vi "thcd_rest_gets.vi"(2 "thcd_delay":u32=500, 3 "thcd_visa":refnum<visa-resource-name>) -> ()   [LabVIEW 2013]
panel:
  in  "thcd_ch":u8(ring) items=["1"=1, "2"=2, "3"=3, "4"=4, "all"=5]
  in  "thcd_com":T1(ring)
  out "error out":errorcluster
  in  "error in":errorcluster
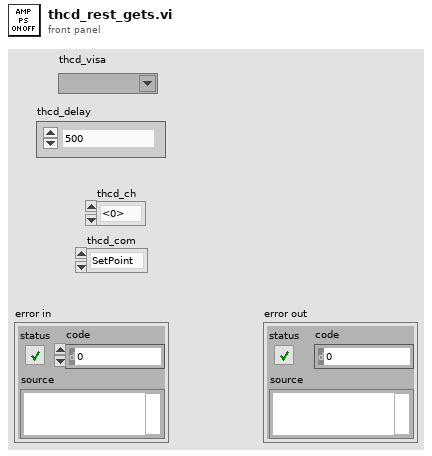
[diagram p1: front panel]
types:
  T1 = enum8{"SetPoint", "AlarmH", "AlarmL", "AlarmHys", "Units", "GasID", "SigInput", "Filter", "Multiplier", "Display", "ReadCh"}
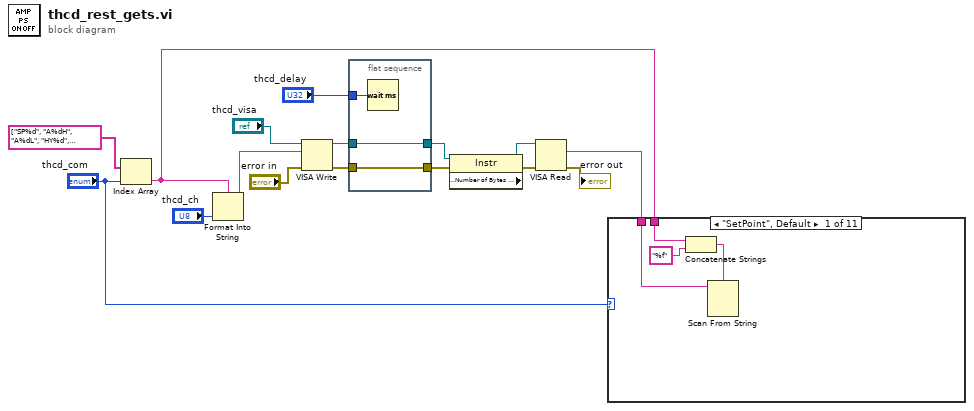
[diagram p0: block diagram]
diagram:
  n1 = Index Array(array=string[] ["SP%d", "A%dH", "A%dL", "HY%d", "UM%d", "GS%d", "IN%d", "FL%d", "ML%d", "D%d", "C%d"] ("Array"), index="thcd_com") -> (element=w1:string)
  n2 = Format Into String(format string=w1, "thcd_ch") -> (resulting string=w5:string)  [unwired: 2 in, 1 out]
  n3 = VISA Write(VISA resource name="thcd_visa", write buffer=w5, error in (no error)="error in") -> (VISA resource name out=w14:refnum<visa-resource-name>, error out=w16:errorcluster)  [unwired: 1 out]
  n4 = flat-sequence {
    tunnel: w16 -> [w18]
    tunnel: [w18] -> w15
    tunnel: w14 -> [w17]
    tunnel: [w17] -> w13
    tunnel: "thcd_delay" -> [w19]
    frame #0 {
      n5 = Wait (ms)(milliseconds to wait=w19) -> ()  [unwired: 1 out]
    }
  }
  n6 = property class="Instr" props=["Serial Settings:Number of Bytes at Serial Port"](reference=w13, error in=w15) -> (reference out=w12:refnum<visa-resource-name>, error out=w11:errorcluster)  [unwired: 1 out]
  n7 = VISA Read(VISA resource name=w12, error in (no error)=w11) -> (read buffer=w2:string, error out=→"error out":errorcluster)  [unwired: 1 in, 2 out]
  n8 = case shown="\"SetPoint\", Default" "thcd_com" {
    tunnel: w2 -> [w23 _ _ _ _ _ _ _ _ _ _]
    tunnel: w1 -> [w22 _ _ _ _ _ _ _ _ _ _]
    frame "SetPoint", Default {
      n9 = Concatenate Strings(w22, "%f" ("string")) -> (w20:string)
      n10 = Scan From String(format string=w20, input string=w23) -> ()  [unwired: 4 in, 3 out]
    }
    frame "AlarmH" {
    }
    frame "AlarmL" {
    }
    frame "AlarmHys" {
    }
    frame "Units" {
    }
    frame "GasID" {
    }
    frame "SigInput" {
    }
    frame "Filter" {
    }
    frame "Multiplier" {
    }
    frame "Display" {
    }
    frame "ReadCh" {
    }
  }
